vi "ts_tree_display_list.vi"(8 "error in (no error)":errorcluster, 10 "ts.list":T1[](array[typedef]), 11 "Tree.in":refnum<vi>) -> (0 "error out":errorcluster, 3 "Tree.out":refnum<vi>)   [LabVIEW 2015]
uses:
  ts-data.ctl
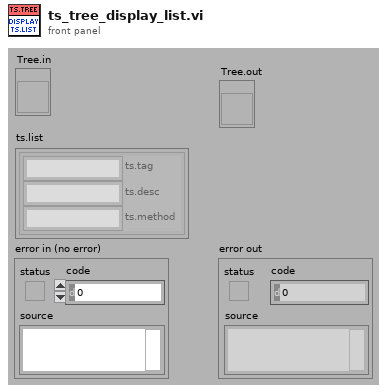
[diagram p1: front panel]
types:
  T1 = typedef "ts-data.ctl" = cluster{"ts.tag":string, "ts.desc":string, "ts.method":string}
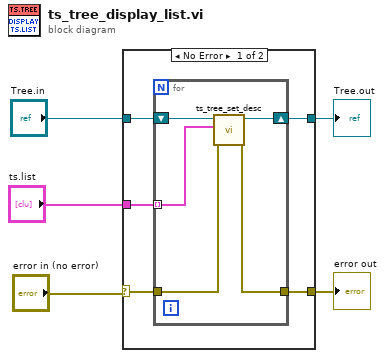
[diagram p0: block diagram]
diagram:
  n1 = case shown="No Error" "error in (no error)" {
    selector: "error in (no error)" -> [w8 w16]
    tunnel: "Tree.in" -> [w10 w17]
    tunnel: [w9 w17] -> w3
    tunnel: [w6 w16] -> w2
    tunnel: "ts.list" -> [w7 _]
    frame No Error {
      n2 = for {
        shift-right: [w11] -> w9
        shift-left: w10 -> [w13]
        tunnel: w8 -> [w15]
        tunnel: w7 -> [w14] mode=indexing
        tunnel: [w12] -> w6
        n3 = call "ts_tree_set_desc.vi"("error in (no error)"=w15, "ts.data"=w14, "Tree.in"=w13) -> ("error out"=w12:errorcluster, "Tree.out"=w11:refnum<vi>)  [unwired: 7 in]
      }
    }
    frame Error {
    }
  }
  "Tree.out" <- w3
  "error out" <- w2
